vi "PowerMonitorType.vi"() -> ()   [LabVIEW 2017]
panel:
  out "Flag_220":bool
  in  "PowerMonitorType":enum16{"DAQ", "MPM_220", "TSL_LOGG"}(ring)
  in  "Product_MPM":enum32{"rdompm210", "rdompm220"}(radio) caption="Product MPM"
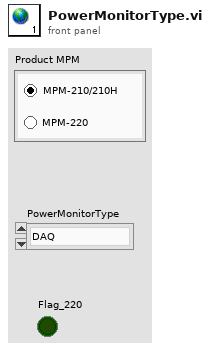
[diagram p1: front panel]
diagram:
